vi "xz.vi"() -> ()   [LabVIEW 2017]
uses:
  <instrlib>/Siglent SDG X Series/Siglent SDG X Series.lvlib
panel:
  in  "VISA resource name":refnum<visa-resource-name>
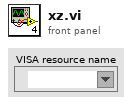
[diagram p1: front panel]
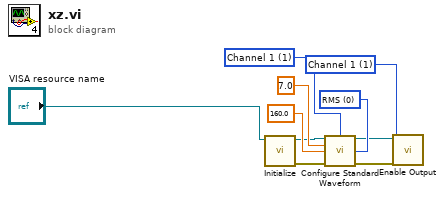
[diagram p0: block diagram]
diagram:
  w2 = 1 items=["Channel 1"=1, "Channel 2"=2] ("Channel (1:Channel 1)")
  w9 = 1 items=["Channel 1"=1, "Channel 2"=2] ("Channel (1:Channel 1)")
  w7 = u16 0 items=["RMS", "pp", "dBm"] ("v-type")
  n1 = call <instrlib>:"Initialize.vi"("VISA resource name"="VISA resource name") -> ("error out"=w6:errorcluster, "VISA resource name out"=w5:refnum<visa-resource-name>)  [unwired: 9 in]
  n2 = call <instrlib>:"Configure Standard Waveform.vi"("VISA resource name"=w5, "Channel (1:Channel 1)"=w9, "Amplitude (1.0 Vpp)"=7.0, "Frequency (1000 Hz)"=160.0, "v-type"=w7, "error in (no error)"=w6) -> ("VISA resource name out"=w3:refnum<visa-resource-name>, "error out"=w4:errorcluster)  [unwired: 8 in]
  n3 = call <instrlib>:"Enable Output.vi"("error in (no error)"=w4, "Channel (1:Channel 1)"=w2, "VISA resource name"=w3) -> ()  [unwired: 7 in, 2 out]
